vi "Switch Configure (7001).vi"(7 "Resistivity":T1, 8 "error in (no error)":errorcluster, 11 "VISA resource name in":refnum<visa-resource-name>) -> (0 "error out":errorcluster, 3 "VISA resource name out":refnum<visa-resource-name>)   [LabVIEW 2016, in "Hall Effect Library.lvlib"]
uses:
  Hall Effect Library.lvlib
  Public/Controls/Resisitivity.ctl
  <instrlib>/Keithley 7001/Keithley 7001.lvlib
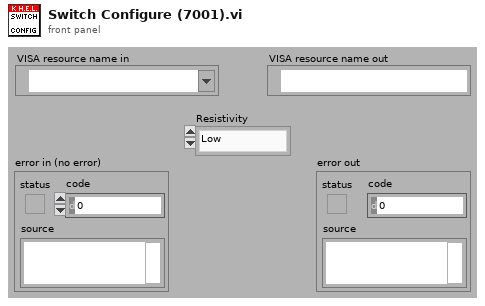
[diagram p1: front panel]
types:
  T1 = typedef "Hall Effect Library.lvlib/Resisitivity.ctl" = enum16{"Low", "High"}
  T2 = enum16{"None", "7052", "7053", "7054", "7056", "7057", "7058", "7059", "7061", "7062", "7063", "7064", "7065", "7066", "7067", "7152", "7153", "7154", "7156", "7158", "7164", "7166", "7168", "7169", "7402", "9990", "9991"}
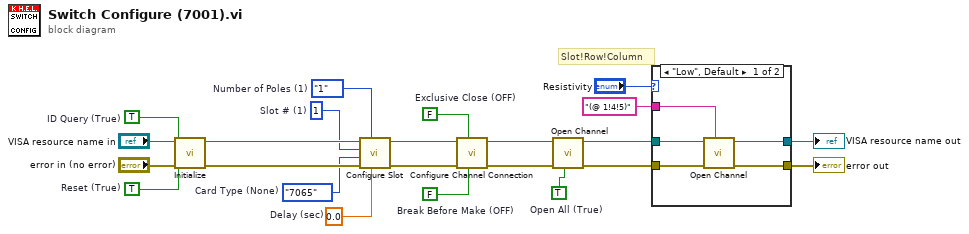
[diagram p0: block diagram]
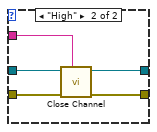
[diagram p2: hidden frame]
diagram:
  w1 = TRUE  # Open All (True)
  w6 = enum16{"1", "2", "4"}."1"  # Number of Poles (1)
  w7 = 0.0  # Delay (sec)
  w8 = T2."7065"  # Card Type (None)
  w9 = TRUE  # Reset (True)
  w10 = TRUE  # ID Query (True)
  w11 = u32 1  # Slot # (1)
  w12 = FALSE  # Break Before Make (OFF)
  w13 = FALSE  # Exclusive Close (OFF)
  # "Slot!Row!Column"
  n1 = call <instrlib>:"Initialize.vi"("error in (no error)"="error in (no error)", "Reset (True)"=w9, "ID Query (True)"=w10, "VISA resource name"="VISA resource name in") -> ("error out"=w16:errorcluster, "VISA resource name out"=w17:refnum<visa-resource-name>)  [unwired: 1 in, 5 out]
  n2 = call <instrlib>:"Configure Slot.vi"("Delay (sec)"=w7, "Number of Poles (1)"=w6, "error in"=w16, "Card Type (None)"=w8, "Slot # (1)"=w11, "VISA resource name"=w17) -> ("error out"=w15:errorcluster, "VISA resource name out"=w14:refnum<visa-resource-name>)  [unwired: 4 out]
  n3 = call <instrlib>:"Configure Channel Connection.vi"("Break Before Make (OFF)"=w12, "Exclusive Close (OFF)"=w13, "error in"=w15, "VISA resource name"=w14) -> ("error out"=w2:errorcluster, "VISA resource name out"=w3:refnum<visa-resource-name>)  [unwired: 6 out]
  n4 = call <instrlib>:"Open Channel.vi"("Open All (False)"=w1, "error in (no error)"=w2, "VISA resource name"=w3) -> ("error out"=w5:errorcluster, "VISA resource name out"=w4:refnum<visa-resource-name>)  [unwired: 1 in, 6 out]
  n5 = case shown="\"Low\", Default" "Resistivity" {
    tunnel: "(@ 1!4!5)" -> [w28 w33]
    tunnel: w4 -> [w25 w32]
    tunnel: w5 -> [w24 w31]
    tunnel: [w26 w30] -> w20
    tunnel: [w27 w29] -> w21
    frame "Low", Default {
      n6 = call <instrlib>:"Open Channel.vi"("Channel List"=w28, "error in (no error)"=w24, "VISA resource name"=w25) -> ("error out"=w26:errorcluster, "VISA resource name out"=w27:refnum<visa-resource-name>)  [unwired: 1 in, 6 out]
    }
    frame "High" {
      n7 = call <instrlib>:"Close Channel.vi"("Channel List"=w33, "error in (no error)"=w31, "VISA resource name"=w32) -> ("error out"=w30:errorcluster, "VISA resource name out"=w29:refnum<visa-resource-name>)  [unwired: 7 out]
    }
  }
  "error out" <- w20
  "VISA resource name out" <- w21
